vi "Wait For Current Play To Finish Core.vi"(9 "Timeout (seconds) (Infinity)":dbl, 11 "Sound Visualizer in":refnum<class "Sound Visualizer.lvclass">) -> (0 "error out":errorcluster, 3 "Sound Visualizer out":refnum<class "Sound Visualizer.lvclass">)   [LabVIEW 2017, in "Sound Visualizer.lvclass"]
doc: "Wait for the sound currently playing on the player to complete. The default time out is \"Infinity\". Wiring a negative value will return an error."
uses:
  Sound Visualizer.lvclass
  Sound Visualizer.lvclass/Sound Visualizer.ctl
  Visualizer/Visualizer.lvlib
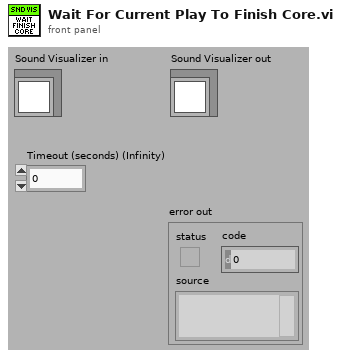
[diagram p1: front panel]
types:
  T1 = typedef "Visualizer.lvlib/Visualizer Type ID.ctl" = u32
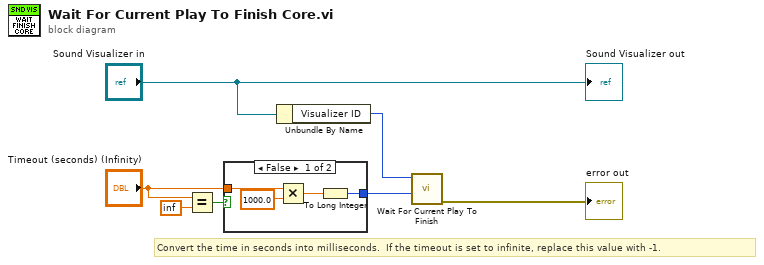
[diagram p0: block diagram]
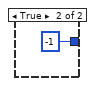
[diagram p2: hidden frame]
diagram:
  # "Convert the time in seconds into milliseconds.  If the timeout is set to infinite, replace this value with -1."
  n1 = Equal?(x="Timeout (seconds) (Infinity)", y=inf) -> (x = y?=w4:bool)
  n2 = case shown="False" w4 {
    tunnel: "Timeout (seconds) (Infinity)" -> [w11 _]
    tunnel: [w8 -1] -> w2
    frame False {
      n3 = Multiply(x=w11, y=1000.0) -> (x*y=w9:dbl)
      n4 = To Long Integer(number=w9) -> (32bit integer=w8:i32)
    }
    frame True {
    }
  }
  n5 = Unbundle By Name("Sound Visualizer in") -> ("Visualizer ID"=w6:T1)
  n6 = call "Wait For Current Play To Finish.vi"("timeout in ms (-1)"=w2, "Visualizer ID"=w6) -> ("error out"=→"error out":errorcluster)  [unwired: 8 in, 1 out]
  "Sound Visualizer out" <- "Sound Visualizer in"
